vi "display.vi"(8 "error in (no error)":errorcluster, 10 "TransactionList.lvclass":refnum<class "TransactionList.lvclass">, 11 "TransactionListUserInterface in":refnum<class "TransactionListUIAdapter.lvclass">) -> (0 "error out":errorcluster, 3 "TransactionListUserInterface out":refnum<class "TransactionListUIAdapter.lvclass">)   [LabVIEW 2018, in "TransactionListUIAdapter.lvclass"]
uses:
  TransactionListUIAdapter.lvclass
  Statement/TransactionList.lvclass
  TransactionListUIAdapter.lvclass/TransactionListUIAdapter.ctl
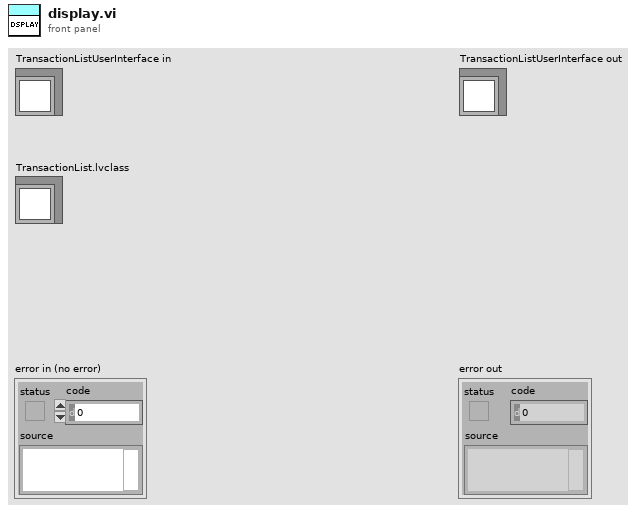
[diagram p1: front panel]
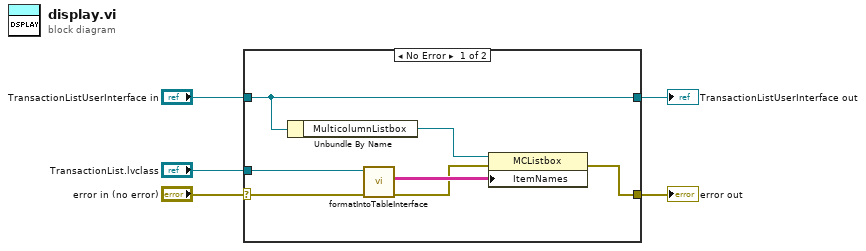
[diagram p0: block diagram]
diagram:
  n1 = case shown="No Error" "error in (no error)" {
    selector: "error in (no error)" -> [w8 w13]
    tunnel: "TransactionList.lvclass" -> [w12 _]
    tunnel: "TransactionListUserInterface in" -> [w7 w14]
    tunnel: [w10 w13] -> w1
    tunnel: [w7 w14] -> w2
    frame No Error {
      n2 = Unbundle By Name(w7) -> ("MulticolumnListbox"=w6:refnum<vi>)
      n3 = call "formatIntoTableInterface.vi"("error in (no error)"=w8, "TransactionList in"=w12) -> ("error out"=w9:errorcluster, "Table Row"=w11:string[][])  [unwired: 7 in, 1 out]
      n4 = property class="MCListbox"(reference=w6, error in=w9, "ItemNames"=w11) -> (error out=w10:errorcluster)  [unwired: 1 out]
    }
    frame Error {
    }
  }
  "error out" <- w1
  "TransactionListUserInterface out" <- w2
